vi "Test Assert Not Equal Value (Typedef).vi"(8 "error in (no error)":errorcluster) -> (0 "error out":errorcluster)   [LabVIEW 2009]
uses:
  <vilib>/picture/picture.llb/imagedata.ctl
  <vilib>/Utility/miscctls.llb/LVBoundsTypeDef.ctl
  classes/Assert/Assert.lvclass
  classes/Test/Test.lvclass
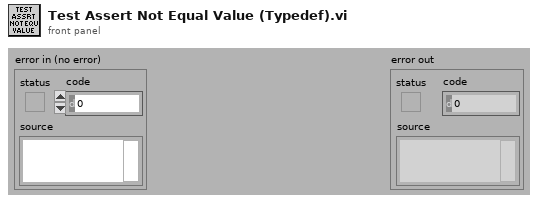
[diagram p1: front panel]
types:
  T1 = typedef "LVBoundsTypeDef.ctl" = cluster{"Width":u32, "Height":u32}
  T2 = cluster{"image type":i32, "image depth":i32, "image":u8[], "mask":u8[], "colors":u32[], "Rectangle":cluster{"left":i16, "top":i16, "right":i16, "bottom":i16}}
  T3 = typedef "imagedata.ctl" = cluster{"image type":i32, "image depth":i32, "image":u8[], "mask":u8[], "colors":u32[], "Rectangle":cluster{"left":i16, "top":i16, "right":i16, "bottom":i16}}
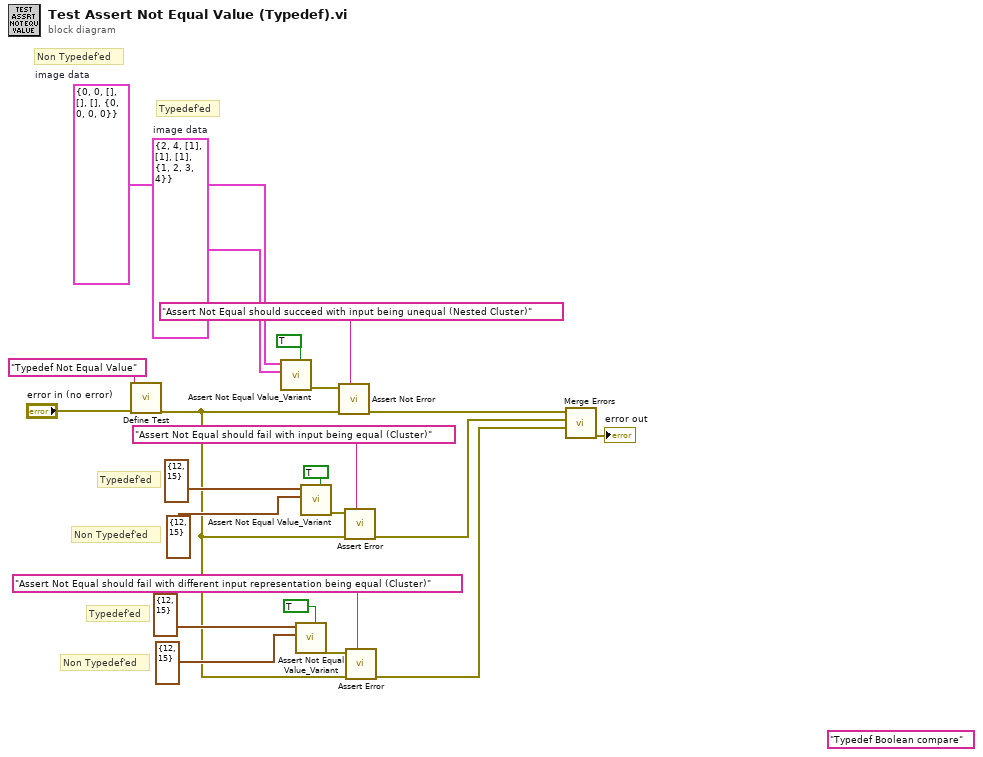
[diagram p0: block diagram]
diagram:
  w11 = T2 {"image type"=0, "image depth"=0, "image"=[], "mask"=[], "colors"=[], "Rectangle"={"left"=0, "top"=0, "right"=0, "bottom"=0}}  # image data
  w10 = T3 {"image type"=2, "image depth"=4, "image"=[1], "mask"=[1], "colors"=[1], "Rectangle"={"left"=1, "top"=2, "right"=3, "bottom"=4}}  # image data
  (unwired) "Typedef Boolean compare" ("Label")
  # "Non Typedef'ed"
  # "Typedef'ed"
  # "Non Typedef'ed"
  # "Typedef'ed"
  # "Non Typedef'ed"
  # "Typedef'ed"
  n1 = call "Define Test.vi"("error in (no error)"="error in (no error)", "Label (VI Title)"="Typedef Not Equal Value") -> ("error out"=w2:errorcluster)  [unwired: 9 in]
  n2 = call "Assert Not Equal Value_Variant.vi"("Assert Only? (F)"=TRUE, "Y"=w10, "X"=w11) -> ("error out"=w17:errorcluster)  [unwired: 8 in]
  n3 = call "Assert Not Equal Value_Variant.vi"("Assert Only? (F)"=TRUE, "Y"=cluster{"Width":u32, "Height":i32} {"Width"=12, "Height"=15} ("Bounds"), "X"=T1 {"Width"=12, "Height"=15} ("Bounds")) -> ("error out"=w3:errorcluster)  [unwired: 8 in]
  n4 = call "Assert Not Equal Value_Variant.vi"("Assert Only? (F)"=TRUE, "Y"=cluster{"Width":u32, "Height":u32} {"Width"=12, "Height"=15} ("Bounds"), "X"=T1 {"Width"=12, "Height"=15} ("Bounds")) -> ("error out"=w15:errorcluster)  [unwired: 8 in]
  n5 = call "Assert Not Error.vi"("Label"="Assert Not Equal should succeed with input being unequal (Nested Cluster)", "error in (no error)"=w2, "Not Error?"=w17) -> ("error out"=w19:errorcluster)  [unwired: 8 in]
  n6 = call "Assert Error.vi"("Label"="Assert Not Equal should fail with input being equal (Cluster)", "error in (no error)"=w2, "Error?"=w15) -> ("error out"=w20:errorcluster)  [unwired: 8 in]
  n7 = call "Assert Error.vi"("Label"="Assert Not Equal should fail with different input representation being equal (Cluster)", "error in (no error)"=w2, "Error?"=w3) -> ("error out"=w1:errorcluster)  [unwired: 8 in]
  n8 = call <vilib>:"Merge Errors.vi"("error in 3 (no error)"=w1, "error in 2 (no error)"=w20, "error in 1 (no error)"=w19) -> ("error out"=→"error out":errorcluster)  [unwired: 4 in]
